vi "CheckAsset.vi"(10 "DataEvent":T6, 11 "Asset":T1) -> (3 "match":bool)   [LabVIEW 2016]
doc: "Determines if the data event belongs to the asset."
uses:
  <vilib>/addons/InsightCM/Utilities/PropertyHelpers/PropertyHelpers.lvlib
  <vilib>/addons/InsightCM/MessageBus/Base/controls/KeyValuePair.ctl
  <vilib>/addons/InsightCM/MessageBus/Base/controls/DataEvent.ctl
  <vilib>/addons/InsightCM/MessageBus/Base/controls/AssetState.ctl
  <vilib>/addons/InsightCM/MessageBus/Base/controls/Metric.ctl
  <vilib>/addons/InsightCM/MessageBus/Base/controls/AssetNodeReference.ctl
  <vilib>/addons/InsightCM/MessageBus/Base/controls/AssetNodeView.ctl
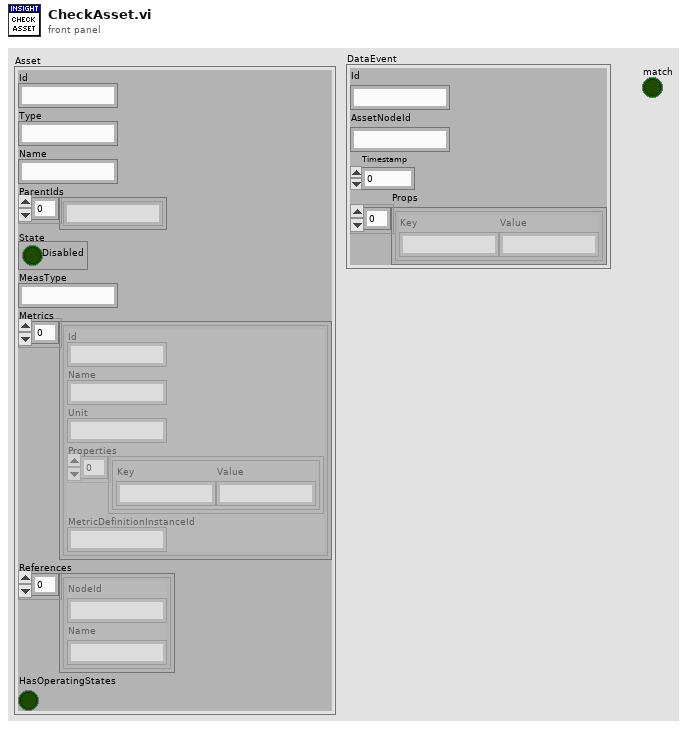
[diagram p1: front panel]
types:
  T1 = typedef "AssetNodeView.ctl" = cluster{"Id":string, "Type":string, "Name":string, "ParentIds":string[], "State":T2, "MeasType":string, "Metrics":T3[], "References":T5[], "HasOperatingStates":bool}
  T2 = typedef "AssetState.ctl" = cluster{"Disabled":bool}
  T3 = typedef "Metric.ctl" = cluster{"Id":string, "Name":string, "Unit":string, "Properties":T4[], "MetricDefinitionInstanceId":string}
  T4 = typedef "KeyValuePair.ctl" = cluster{"Key":string, "Value":string}
  T5 = typedef "AssetNodeReference.ctl" = cluster{"NodeId":string, "Name":string}
  T6 = typedef "DataEvent.ctl" = cluster{"Id":string, "AssetNodeId":string, "Timestamp":i64, "Props":T4[]}
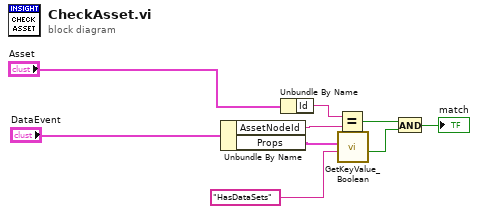
[diagram p0: block diagram]
diagram:
  n1 = Unbundle By Name("DataEvent") -> ("AssetNodeId"=w8:string, "Props"=w7:T4[])
  n2 = Unbundle By Name("Asset") -> ("Id"=w9:string)
  n3 = Equal?(x=w9, y=w8) -> (x = y?=w3:bool)
  n4 = call <vilib>:"GetKeyValue_Boolean.vi"("key"="HasDataSets", "key value pairs"=w7) -> ("value"=w2:bool)  [unwired: 7 in, 2 out]
  n5 = And(x=w3, y=w2) -> (x .and. y?=→"match":bool)
